vi "Build Async Parameters.vi"(8 "Error in":errorcluster, 11 "CompiledSettings In":T1 {"Result Ch Data Refs" format="%.0x"; "Parameter Block Data Refs"."Data Reference" format="%.0x"}) -> (0 "Error out":errorcluster, 2 "Async State Vars":T5, 3 "CompiledSettings Out":T1 {"Result Ch Data Refs" format="%.0x"; "Parameter Block Data Refs"."Data Reference" format="%.0x"})   [LabVIEW 2017, in "Waveform-Processing-Custom-Device Engine.lvlib"]
uses:
  Waveform-Processing-Custom-Device Engine.lvlib
  Types/AsyncStateVariables.ctl
  <vilib>/NI VeriStand/Custom Device Waveform API/Single Waveform Read (DBL)/Single Waveform Read (DBL).lvclass
  <vilib>/NI VeriStand/Custom Device Waveform API/Single Waveform Write (DBL)/Single Waveform Write (DBL).lvclass
  <vilib>/NI Veristand/Custom Device API/Waveform Data Reference.ctl
  Types/New Async FIFOs.ctl
  <vilib>/NI/NIVS Inline Async API/_Data Access Engine/Data Access Engine/Types/Write.DVR.ctl
  <vilib>/NI/NIVS Inline Async API/_Data Access Engine/Access Type Classes/Write/Write.lvclass
  Shared/CompiledSettings.ctl
  <vilib>/NI Veristand/Custom Device API/Block Data Reference.ctl
  <vilib>/NI Veristand/Custom Device API/Data Reference.ctl
  <vilib>/NI Veristand/Custom Device API/Custom Device API.lvlib
  <vilib>/NI/NIVS Inline Async API/_Data Access Engine/Data Access Engine/Data Access Engine.lvclass
  Shared/Waveform-Processing-Custom-Device Shared.lvlib
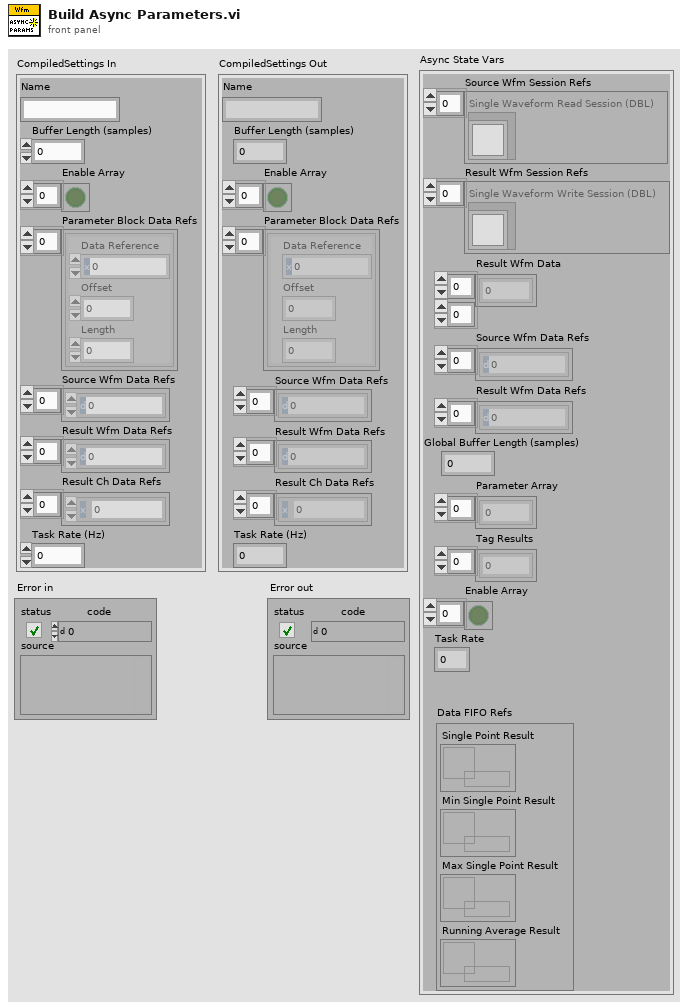
[diagram p1: front panel]
types:
  T1 = typedef "Waveform-Processing-Custom-Device Shared.lvlib/CompiledSettings.ctl" = cluster{"Name":string, "Buffer Length (samples)":u32, "Enable Array":bool[], "Parameter Block Data Refs":T2[], "Source Wfm Data Refs":T4[], "Result Wfm Data Refs":T4[], "Result Ch Data Refs":T3[], "Task Rate (Hz)":dbl}
  T2 = typedef "Custom Device API.lvlib/Block Data Reference.ctl" = cluster{"Data Reference":T3, "Offset":u64, "Length":u64}
  T3 = typedef "Custom Device API.lvlib/Data Reference.ctl" = i32
  T4 = typedef "Custom Device API.lvlib/Waveform Data Reference.ctl" = i32
  T5 = typedef "Waveform-Processing-Custom-Device Engine.lvlib/AsyncStateVariables.ctl" = cluster{"Source Wfm Session Refs":refnum<class "Single Waveform Read (DBL).lvclass">[], "Result Wfm Session Refs":refnum<class "Single Waveform Write (DBL).lvclass">[], "Result Wfm Data":dbl[][], "Source Wfm Data Refs":T4[], "Result Wfm Data Refs":T4[], "Global Buffer Length (samples)":dbl, "Parameter Array":dbl[], "Tag Results":dbl[], "Enable Array":bool[], "Task Rate":dbl, "Data FIFO Refs":T6}
  T6 = typedef "Waveform-Processing-Custom-Device Engine.lvlib/New Async FIFOs.ctl" = cluster{"Single Point Result":T7, "Running Average Result":T7, "Min Single Point Result":T7, "Max Single Point Result ":T7}
  T7 = typedef "Data Access Engine.lvlib/Data Access Engine.lvclass/Write.DVR.ctl" = refnum<data-value>
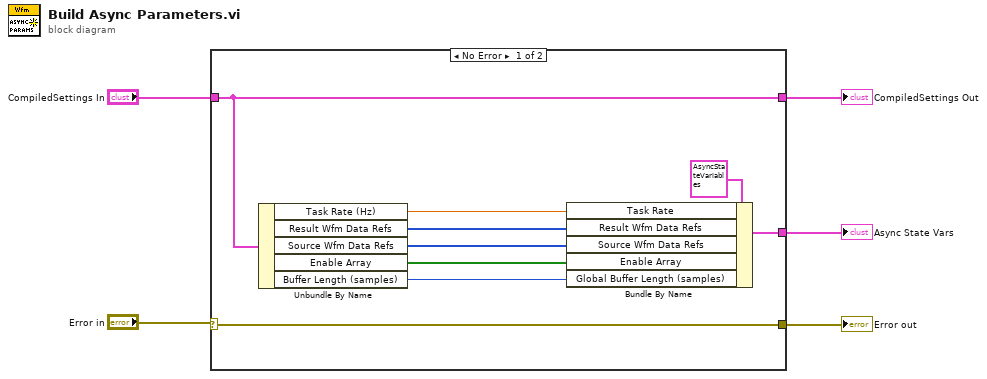
[diagram p0: block diagram]
diagram:
  n1 = case shown="No Error" "Error in" {
    selector: "Error in" -> [w12 w16]
    tunnel: [w12 w16] -> w4
    tunnel: "CompiledSettings In" -> [w13 w15]
    tunnel: [w13 w15] -> w2
    tunnel: [w14 _] -> w1
    frame No Error {
      n2 = Unbundle By Name(w13) -> ("Task Rate (Hz)"=w6:dbl, "Result Wfm Data Refs"=w11:T4[], "Source Wfm Data Refs"=w10:T4[], "Enable Array"=w9:bool[], "Buffer Length (samples)"=w8:u32)
      n3 = Bundle By Name(cluster=T5 {"Source Wfm Session Refs"=[], "Result Wfm Session Refs"=[], "Result Wfm Data"=[], "Source Wfm Data Refs"=[], "Result Wfm Data Refs"=[], "Global Buffer Length (samples)"=0.0, "Parameter Array"=[], "Tag Results"=[], "Enable Array"=[], "Task Rate"=0.0, "Data FIFO Refs"={"Single Point Result"=refnum, "Running Average Result"=refnum, "Min Single Point Result"=refnum, "Max Single Point Result "=refnum}} ("Async State Vars 2"), "Task Rate"=w6, "Result Wfm Data Refs"=w11, "Source Wfm Data Refs"=w10, "Enable Array"=w9, "Global Buffer Length (samples)"=w8) -> (w14:T5)
    }
    frame Error {
    }
  }
  "Error out" <- w4
  "Async State Vars" <- w1
  "CompiledSettings Out" <- w2
